vi "MultiStation@Blinking__Parameter.vi"(1 "ParamterIn":string) -> (0 "ParamterOut":string)   [LabVIEW 2019]
panel:
  in  "IDName":string(combo)
  in  "Parameter":string(combo)
  in  "StationName":string(combo)
  in  "Confirm":bool
  # "MultiStation@General $Station.$ID(,ParameterS)"
  # "."
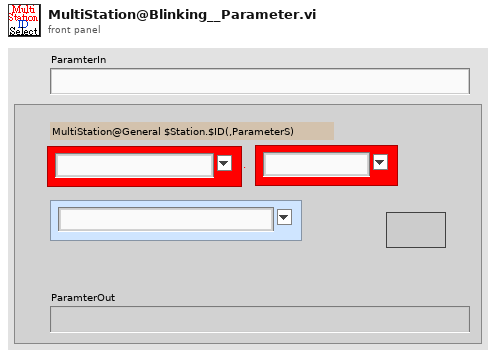
[diagram p1: front panel]
types:
  T1 = enum16{"Init", "AddStation", "StateShift", "ResetDefault", "SetStationON", "SetStationOFF", "SetStationOK", "SetStationNG", "UpdateIndicator", "SetData", "GetData", "GetOnOff", "GetOkNg", "ShowFeedInTray", "ShowFeedOutTray", "BlinkingOn", "BlinkingOff"}
  T2 = cluster{"轉盤燈號":refnum<vi>[], "各站資料":cluster{"轉盤燈號":bool, "錯誤燈號":bool, "資料":variant}[], "IDList":string[]}[]
  T3 = cluster{"轉盤燈號":refnum<vi>[], "各站資料":cluster{"轉盤燈號":bool, "錯誤燈號":bool, "資料":variant}[], "IDList":string[]}
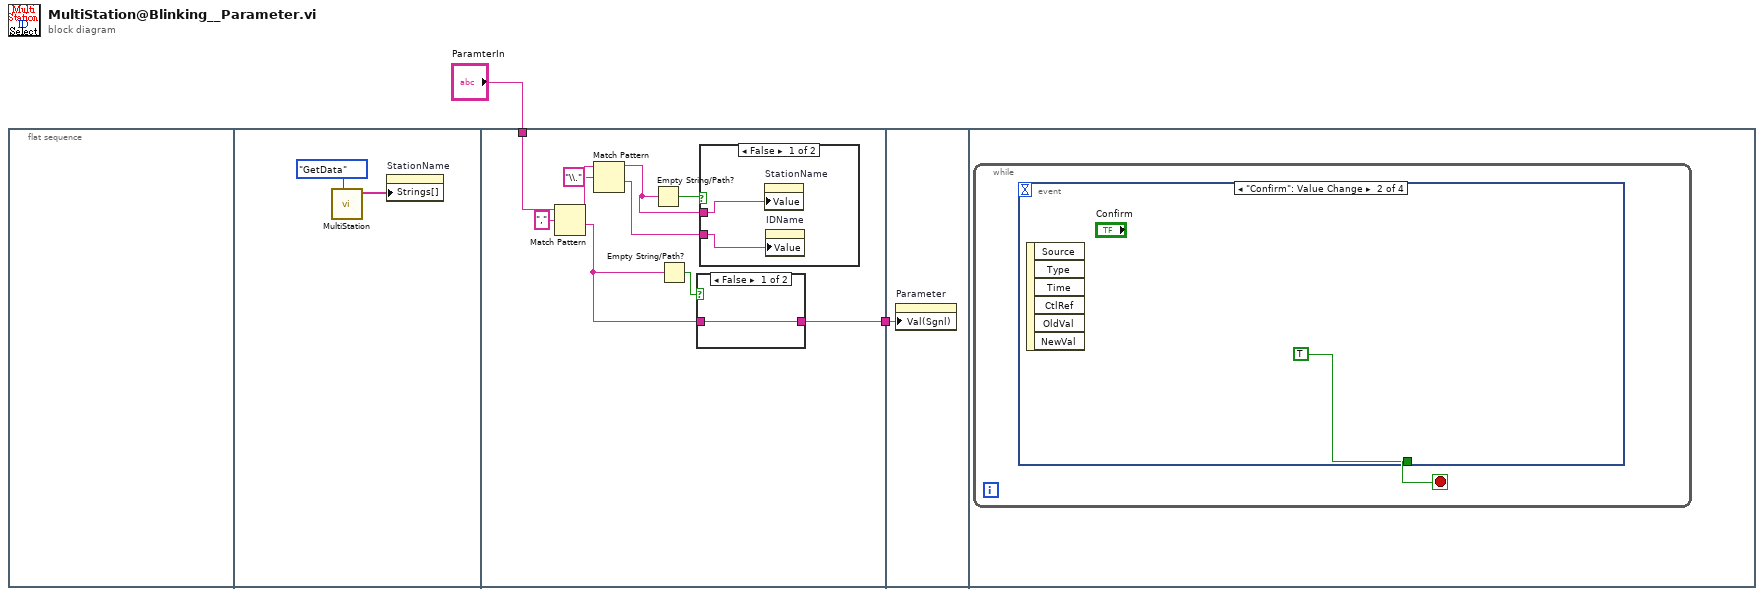
[diagram p0: block diagram]
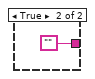
[diagram p2: hidden frame]
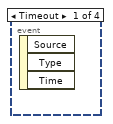
[diagram p4: hidden frame]
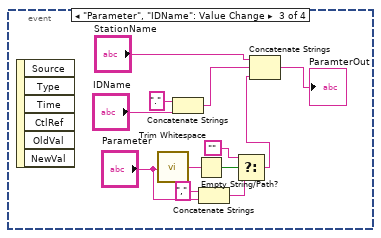
[diagram p5: hidden frame]
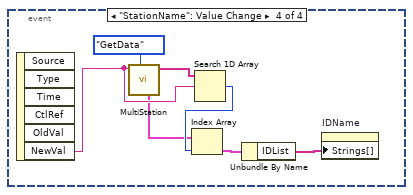
[diagram p6: hidden frame]
diagram:
  n1 = flat-sequence {
    tunnel: "ParamterIn" -> [w11]
    tunnel: [w12] -> w1
    tunnel: w1 -> [w19]
    frame #0 {
    }
    frame #1 {
      n2 = call "MultiStation.vi"("OP"=T1."GetData") -> ("StationList"=w3:string[])  [unwired: 6 in, 4 out]
      n3 = property on="StationName" class="CmbBox"("Strings[]"=w3) -> ()  [unwired: 2 in, 2 out]
    }
    frame #2 {
      n4 = Match Pattern(string=w11, regular expression="," ("search string")) -> (before substring=w8:string, after substring=w9:string)  [unwired: 1 in, 2 out]
      n5 = Match Pattern(string=w8, regular expression="\\.") -> (before substring=w6:string, after substring=w5:string)  [unwired: 1 in, 2 out]
      n6 = Empty String/Path?(string/path=w6) -> (empty?=w14:bool)
      n7 = Empty String/Path?(string/path=w9) -> (empty?=w13:bool)
      n8 = case shown="False" w13 {
        tunnel: [w15 ""] -> w12
        tunnel: w9 -> [w15 _]
        frame False {
        }
        frame True {
        }
      }
      n9 = case shown="False" w14 {
        tunnel: w6 -> [w18 _]
        tunnel: w5 -> [w17 _]
        frame False {
          n10 = property on="StationName" class="CmbBox"("Value"=w18) -> ()  [unwired: 2 in, 2 out]
          n11 = property on="IDName" class="CmbBox"("Value"=w17) -> ()  [unwired: 2 in, 2 out]
        }
        frame True {
        }
      }
    }
    frame #3 {
      n12 = property on="Parameter" class="CmbBox"("Val(Sgnl)"=w19) -> ()  [unwired: 2 in, 2 out]
    }
    frame #4 {
      n13 = while {
        stop <- w20 stop-if-true
        n14 = event shown="[1] \"Confirm\": Value Change" {
          selector: _ -> [_ _ _ _]
          dyn-events: _ -> [_ _ _ _]
          timeout: _ -> [_ _ _ _]
          tunnel: [_ TRUE _ _] -> w20
          event Timeout {
            n15 = event-data() -> ()  [unwired: 1 in, 3 out]
          }
          event "Confirm": Value Change {
            n16 = event-data() -> ()  [unwired: 1 in, 6 out]
          }
          event "Parameter", "IDName": Value Change {
            n17 = event-data() -> ()  [unwired: 1 in, 6 out]
            n18 = call <vilib>:"Trim Whitespace.vi"("string"="Parameter") -> ("trimmed string"=w28:string)  [unwired: 1 in]
            n19 = Concatenate Strings("." ("string"), "IDName") -> (w22:string)
            n20 = Empty String/Path?(string/path=w28) -> (empty?=w29:bool)
            n21 = Concatenate Strings("," ("string"), "Parameter") -> (w31:string)
            n22 = Select(t="", s=w29, f=w31) -> (s? t:f=w25:string)
            n23 = Concatenate Strings("StationName", w22, w25) -> (→"ParamterOut":string)
          }
          event "StationName": Value Change {
            n24 = event-data() -> ("NewVal"=w38:string)  [unwired: 1 in, 5 out]
            n25 = call "MultiStation.vi"("OP"=T1."GetData", "StationID"=w38) -> ("StationList"=w39:string[], "StationInfoS"=w36:T2)  [unwired: 5 in, 3 out]
            n26 = Search 1D Array(1D array=w39, element=w38) -> (index of element=w37:i32)  [unwired: 1 in]
            n27 = Index Array(array=w36, index=w37) -> (element=w35:T3)
            n28 = Unbundle By Name(w35) -> ("IDList"=w34:string[])
            n29 = property on="IDName" class="CmbBox"("Strings[]"=w34) -> ()  [unwired: 2 in, 2 out]
          }
        }
      }
    }
  }
